vi "Record.vi"(8 "error in (no error)":errorcluster, 10 "Waveform":waveform(dbl)[](array[waveform]), 11 "Task_Abstr in":refnum<class "Task_Abstr.lvclass">) -> (0 "error out":errorcluster, 3 "Task_Abstr out":refnum<class "Task_Abstr.lvclass">)   [LabVIEW 2025, in "Task_Abstr.lvlib" / "Task_Abstr.lvclass"]
uses:
  Task_Abstr.lvclass
  <vilib>/Utility/miscctls.llb/LVMapReplaceAction.ctl
  <vilib>/Waveform/WDTOps.llb/WDT Append Waveforms DBL.vi
  Task_Abstr.lvclass/Task_Abstr.ctl
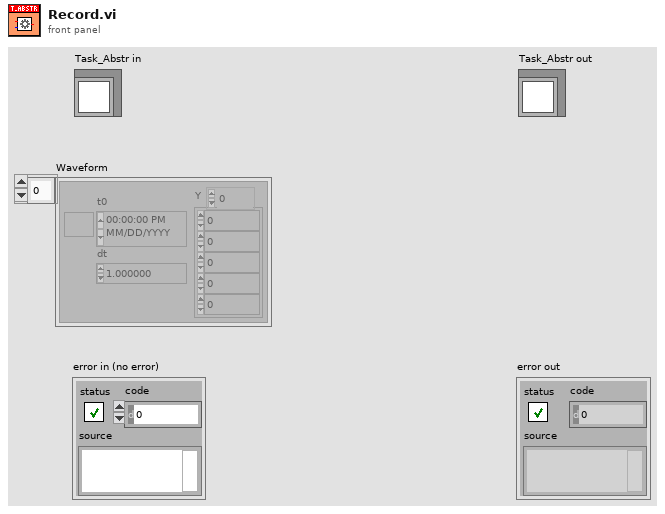
[diagram p1: front panel]
types:
  T1 = typedef "LVMapReplaceAction.ctl" = enum32{"Modify Entry only if found", "Add or Modify Entry", "Delete Entry"}
  T2 = typedef "Task_Abstr.lvlib/Task_Abstr.lvclass/DataContainer.ctl" = map{string, T3}
  T3 = typedef "Task_Abstr.lvlib/Task_Abstr.lvclass/WaveformData.ctl" = cluster{"StartTime":timestamp, "StopTime":timestamp, "Waveform":waveform(dbl)[]}
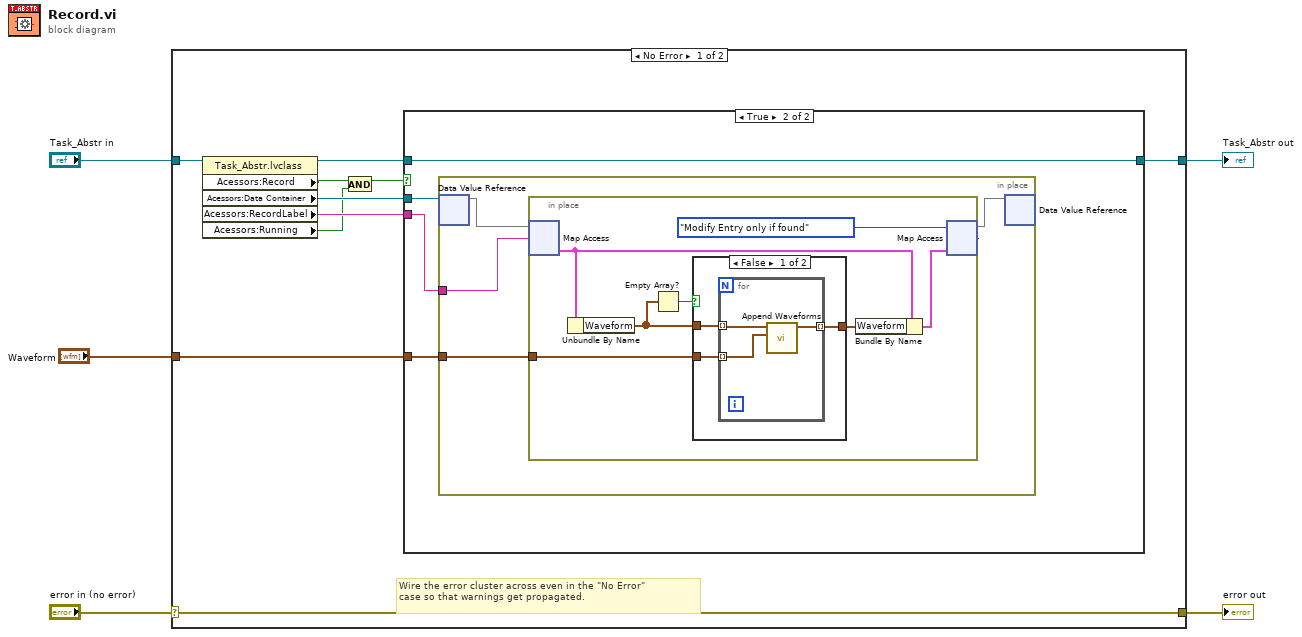
[diagram p0: block diagram]
diagram:
  n1 = case shown="No Error" "error in (no error)" {
    selector: "error in (no error)" -> [w14 w40]
    tunnel: [w14 w40] -> w4
    tunnel: [w11 w39] -> w2
    tunnel: "Task_Abstr in" -> [w15 w39]
    tunnel: "Waveform" -> [w8 _]
    frame No Error {
      # "Wire the error cluster across even in the \"No Error\"\ncase so that warnings get propagated."
      n2 = property class="Task_Abstr.lvclass"(reference=w15) -> (reference out=w12:refnum<class "Task_Abstr.lvclass">, "Acessors:Record"=w13:bool, "Acessors:Data Container"=w10:refnum<data-value>, "Acessors:RecordLabel"=w9:string, "Acessors:Running"=w6:bool)  [unwired: 1 in, 1 out]
      n3 = And(x=w13, y=w6) -> (x .and. y?=w7:bool)
      n4 = case shown="True" w7 {
        tunnel: w12 -> [w16 w20]
        tunnel: [w16 w20] -> w11
        tunnel: w10 -> [_ w17]
        tunnel: w9 -> [_ w19]
        tunnel: w8 -> [_ w18]
        frame False {
        }
        frame True {
          n5 = in-place {
            in-place-border: w19 -> [w24]
            in-place-border: w18 -> [w23]
            n6 = in-place-dvr #1(w17) -> (w22:T2)  [unwired: 1 out]
            n7 = in-place {
              in-place-border: w23 -> [w28]
              n8 = in-place-map #2(w22, w24) -> (w30:T3)  [unwired: 1 in, 1 out]
              n9 = Unbundle By Name(w30) -> ("Waveform"=w26:waveform(dbl)[])
              n10 = Empty Array?(array=w26) -> (empty?=w25:bool)
              n11 = case shown="False" w25 {
                tunnel: w28 -> [w34 w38]
                tunnel: [w33 w38] -> w27
                tunnel: w26 -> [w32 _]
                frame False {
                  n12 = for {
                    tunnel: w32 -> [w37] mode=indexing
                    tunnel: w34 -> [w36] mode=indexing
                    tunnel: [w35] -> w33 mode=indexing
                    n13 = call-poly <vilib>:"Append Waveforms.vi"("waveform B"=w36, "waveform A"=w37) -> ("waveform out"=w35:waveform(dbl))  [unwired: 8 in, 1 out]
                  }
                }
                frame True {
                }
              }
              n14 = Bundle By Name(cluster=w30, "Waveform"=w27) -> (w29:T3)
              n15 = in-place-map #2(w29, LVMapReplaceAction."Modify Entry only if found" ("action")) -> (w21:T2)  [unwired: 2 out]
            }
            n16 = in-place-dvr #1(w21) -> ()  [unwired: 2 out]
          }
        }
      }
    }
    frame Error {
    }
  }
  "error out" <- w4
  "Task_Abstr out" <- w2
